vi "Plot menu selection.vi"(5 "Location":T1, 7 "VI ref":refnum<vi>, 8 "error in (no error)":errorcluster, 9 "ItemPath":string, 10 "ItemTag":string, 11 "BluePlotHandle in":refnum<class "RocketPlotHandle.lvclass">) -> (0 "error out":errorcluster, 3 "BluePlotHandle out":refnum<class "RocketPlotHandle.lvclass">)   [LabVIEW 2021, in "RocketPlotHandle.lvclass"]
uses:
  RocketPlotHandle.lvclass
  TypeDefs/Shortcut Location.ctl
  SubVIs/menu/Plot menu activation submenu type v2.ctl
  TypeDefs/Plot axis.ctl
  RocketPlot.lvlib
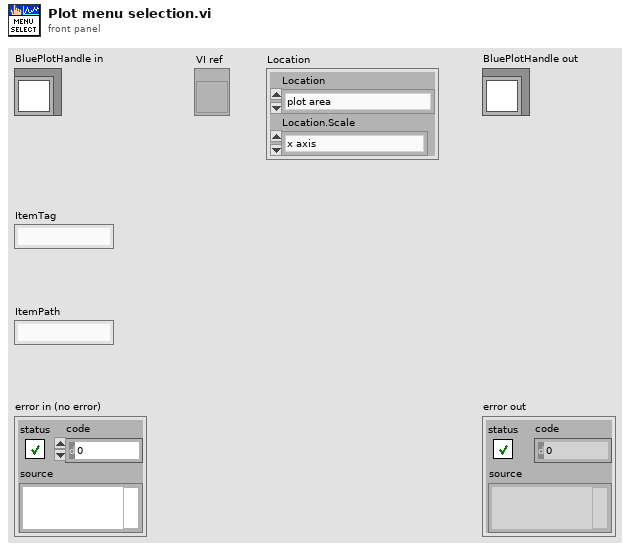
[diagram p1: front panel]
types:
  T1 = typedef "RocketPlot.lvlib/Shortcut Location.ctl" = cluster{"Location":T2, "Location.Scale":T3}
  T2 = typedef "RocketPlot.lvlib/Plot menu activation submenu type v2.ctl" = enum16{"plot area", "plot border", "markers", "scale"}
  T3 = typedef "RocketPlot.lvlib/Plot axis.ctl" = enum16{"x axis", "left axis", "right axis"}
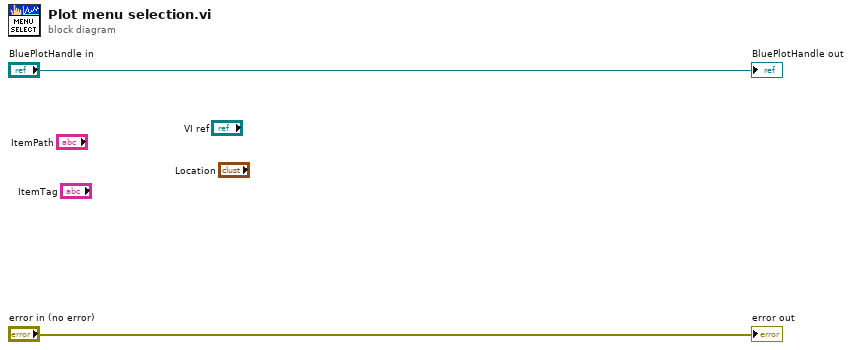
[diagram p0: block diagram]
diagram:
  "error out" <- "error in (no error)"
  "BluePlotHandle out" <- "BluePlotHandle in"
